vi "get data.vi"(8 "error in (no error)":errorcluster, 11 "LineCCD in":refnum<class "LineCCD.lvclass">) -> (0 "error out":errorcluster, 3 "LineCCD out":refnum<class "LineCCD.lvclass">)   [LabVIEW 2012, in "LineCCD.lvclass"]
uses:
  LineCCD.lvclass
  LineCCD.lvclass/LineCCD.ctl
  <instrlib>/ALPHALAS CCD S Series/ALPHALAS CCD S Series.lvlib
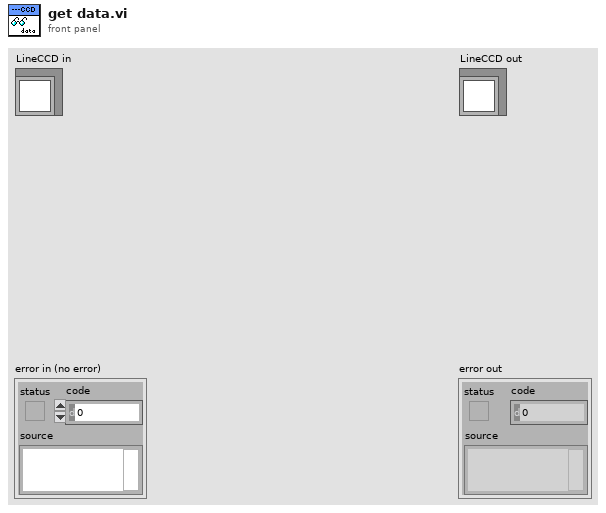
[diagram p1: front panel]
types:
  T1 = typedef "ALPHALAS CCD S Series.lvlib/Operating Mode.ctl" = u16
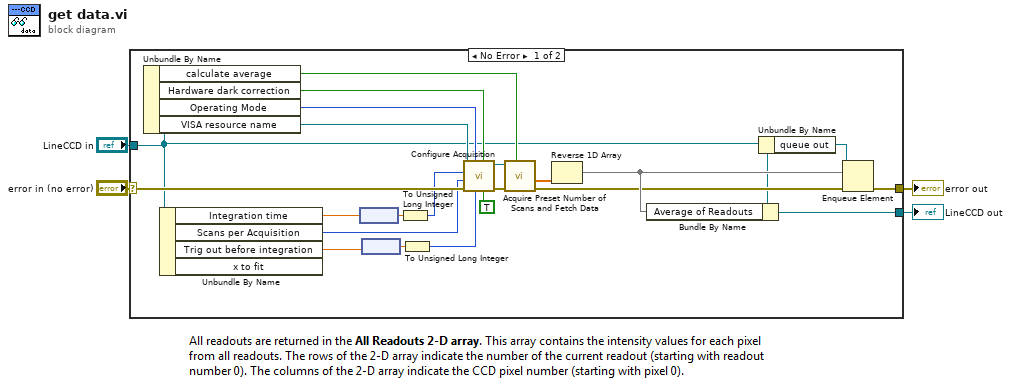
[diagram p0: block diagram]
diagram:
  n1 = case shown="No Error" "error in (no error)" {
    selector: "error in (no error)" -> [w25 w28]
    tunnel: [w10 w28] -> w3
    tunnel: [w26 w27] -> w1
    tunnel: "LineCCD in" -> [w6 w27]
    frame No Error {
      n2 = Unbundle By Name(w6) -> ("calculate average"=w16:bool, "Hardware dark correction"=w14:bool, "Operating Mode"=w15:T1, "VISA resource name"=w22:refnum<visa-resource-name>)
      n3 = Unbundle By Name(w6) -> ("Integration time"=w21:dbl[unit], "Scans per Acquisition"=w12:u32, "Trig out before integration"=w18:dbl[unit])  [unwired: 1 out]
      n4 = node(w21) -> (w20:dbl)
      n5 = node(w18) -> (w19:dbl)
      n6 = To Unsigned Long Integer(number=w20) -> (unsigned 32bit integer=w13:u32)
      n7 = To Unsigned Long Integer(number=w19) -> (unsigned 32bit integer=w11:u32)
      n8 = call <instrlib>:"Configure Acquisition.vi"("Enable Trig Out After Configuration (T: Enabled)"=TRUE, "Hardware Dark Correction (F: Disabled)"=w14, "Trig Out Before Integration (0 µs)"=w11, "Operating Mode (0: Int Synch, Continuously Running w SW Capture-Start)"=w15, "error in (no error)"=w25, "Scans per Acquisition (1)"=w12, "Integration Time (5000 µs)"=w13, "VISA resource name"=w22) -> ("error out"=w24:errorcluster, "VISA resource name out"=w23:refnum<visa-resource-name>)  [unwired: 2 in]
      n9 = call <instrlib>:"Acquire Preset Number of Scans and Fetch Data.vi"("Calculate Average (T: On)"=w16, "error in (no error)"=w24, "VISA resource name"=w23) -> ("error out"=w7:errorcluster, "Average of Readouts"=w5:dbl[])  [unwired: 5 in, 2 out]
      n10 = Reverse 1D Array(array=w5) -> (reversed array=w8:dbl[])
      n11 = Bundle By Name(cluster=w6, "Average of Readouts"=w8) -> (w26:refnum<class "LineCCD.lvclass">)
      n12 = Unbundle By Name(w6) -> ("queue out"=w9:refnum<queue>)
      n13 = Enqueue Element(queue=w9, element=w8, error in (no error)=w7) -> (error out=w10:errorcluster)  [unwired: 1 in, 2 out]
    }
    frame Error {
    }
  }
  "error out" <- w3
  "LineCCD out" <- w1
